vi "Client.vi"() -> ()   [LabVIEW 2025]
uses:
  <vilib>/Utility/miscctls.llb/LVPointTypeDef.ctl
  common/types/network/FieldData.ctl
  common/types/network/FoggedFieldCell.ctl
  server/types/TerrainEnum.ctl
  <vilib>/Utility/miscctls.llb/LVMapReplaceAction.ctl
  2d6ff062-9b47-4ee0-9ab3-b22f700b8ac0.vi
  ClientGlobalVariables.vi
panel:
  out "Network Ready":bool
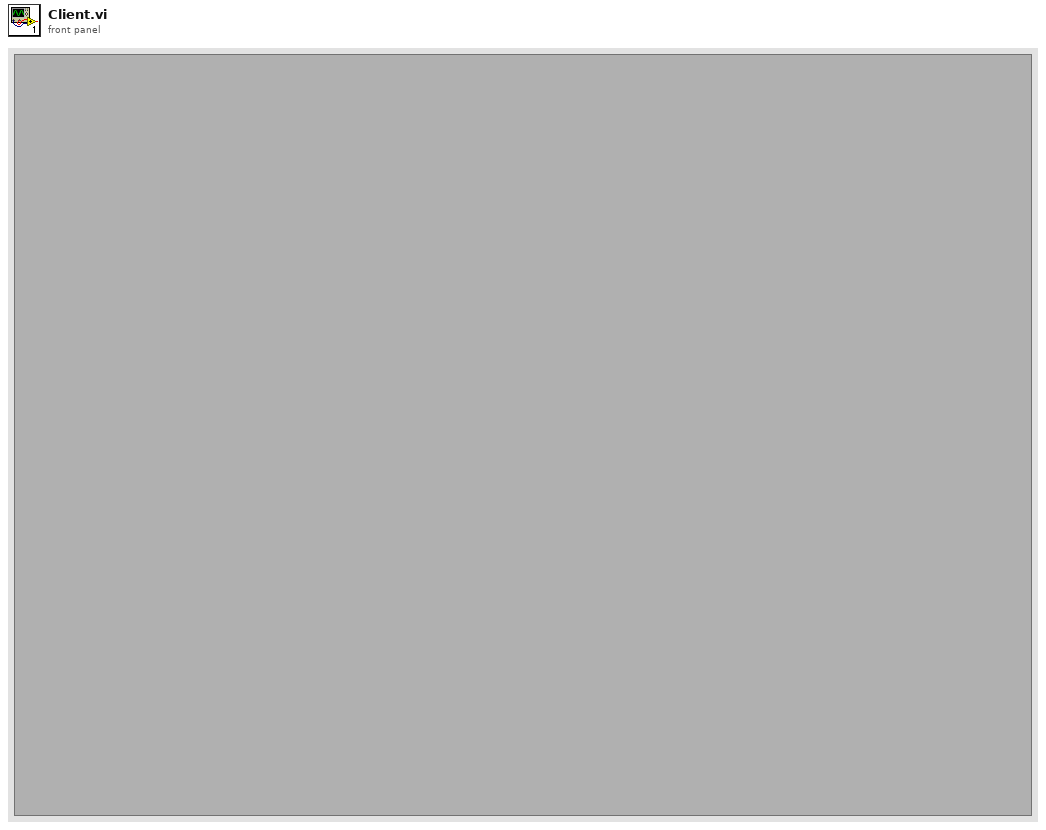
[diagram p1: front panel]
types:
  T1 = cluster{"seconds since 1Jan1904":timestamp, "Data":string}
  T2 = typedef "LVPointTypeDef.ctl" = cluster{"Horizontal":i16, "Vertical":i16}
  T3 = enum16{"Initalize", "Start Menu", "Lobby Menu", "In Game"}
  T4 = cluster{"Action":string, "seconds since 1Jan1904":timestamp, "Data":string}
  T5 = typedef "FieldData.ctl" = cluster{"Round":u32, "FoggedFieldArray":T6[][]}
  T6 = typedef "FoggedFieldCell.ctl" = cluster{"Troops":u32, "Owner":i32, "Terrain":T7, "Fog":bool}
  T7 = typedef "TerrainEnum.ctl" = enum16{"Plain", "Mountain", "City", "General"}
  T8 = map{u32, cluster{"Name":string, "Team":u8, "Ready":bool, "Host":bool, "Alive":bool, "Color":u32, "Lands":set{cluster{"Row":u32, "Column":u32}}, "Army":u32}}
  T9 = cluster{"Name":string, "Team":u8, "Ready":bool, "Host":bool, "Alive":bool, "Color":u32, "Lands":set{cluster{"Row":u32, "Column":u32}}, "Army":u32}
  T10 = typedef "LVMapReplaceAction.ctl" = enum32{"Modify Entry only if found", "Add or Modify Entry", "Delete Entry"}
  T11 = cluster{"ID":u32, "Name":string, "Team":u8, "Ready":bool, "Host":bool, "Alive":bool, "Color":u32, "Lands":set{cluster{"Row":u32, "Column":u32}}, "Army":u32}[]
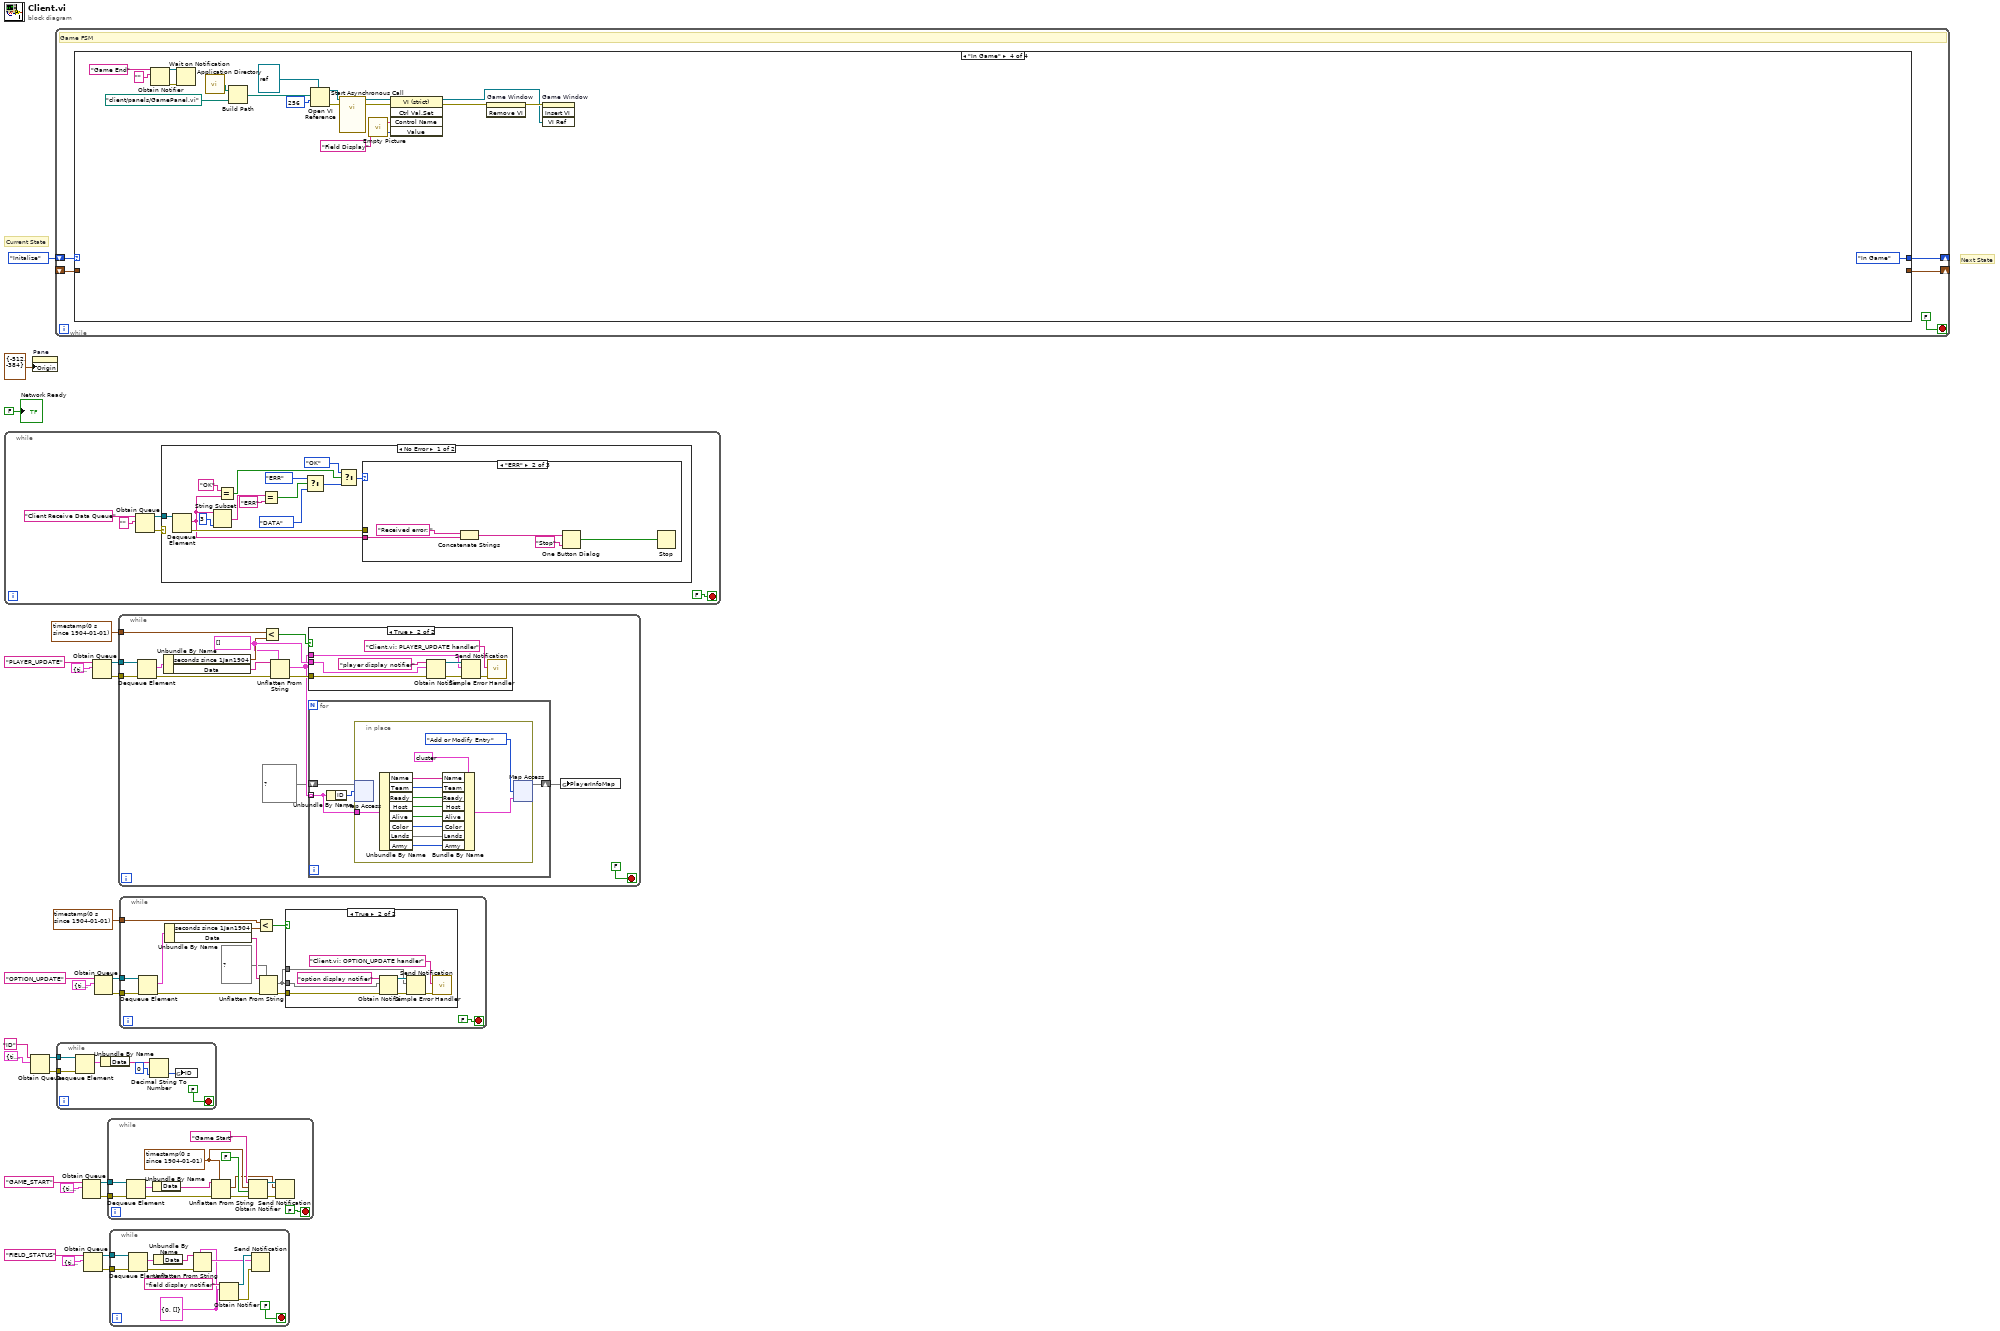
[diagram p0: block diagram]
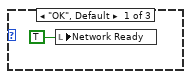
[diagram p4: hidden frame]
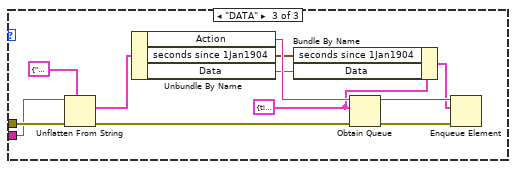
[diagram p5: hidden frame]
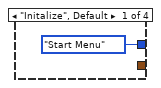
[diagram p7: hidden frame]
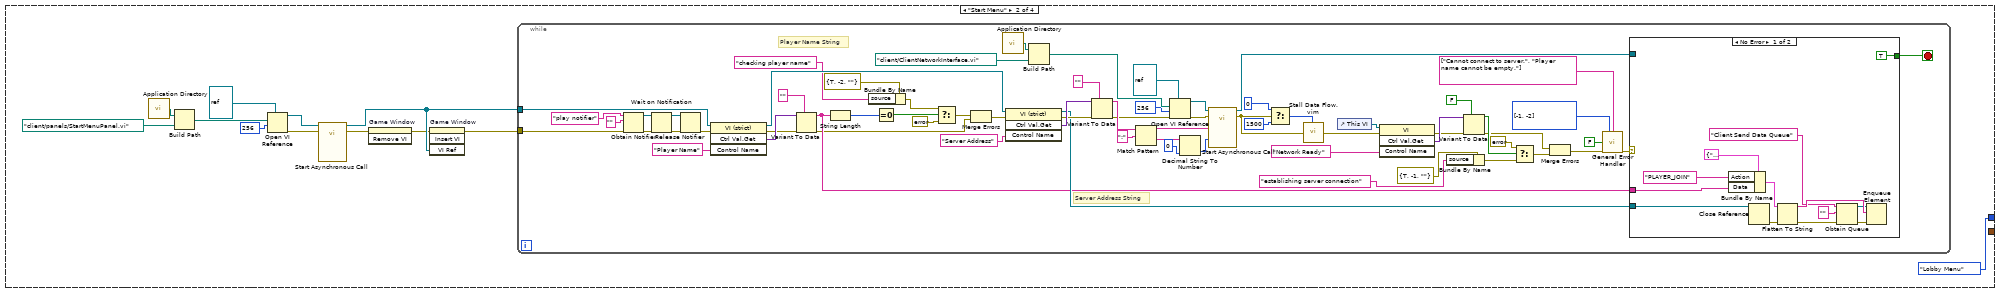
[diagram p8: hidden frame]
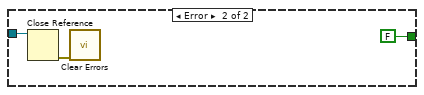
[diagram p9: hidden frame]
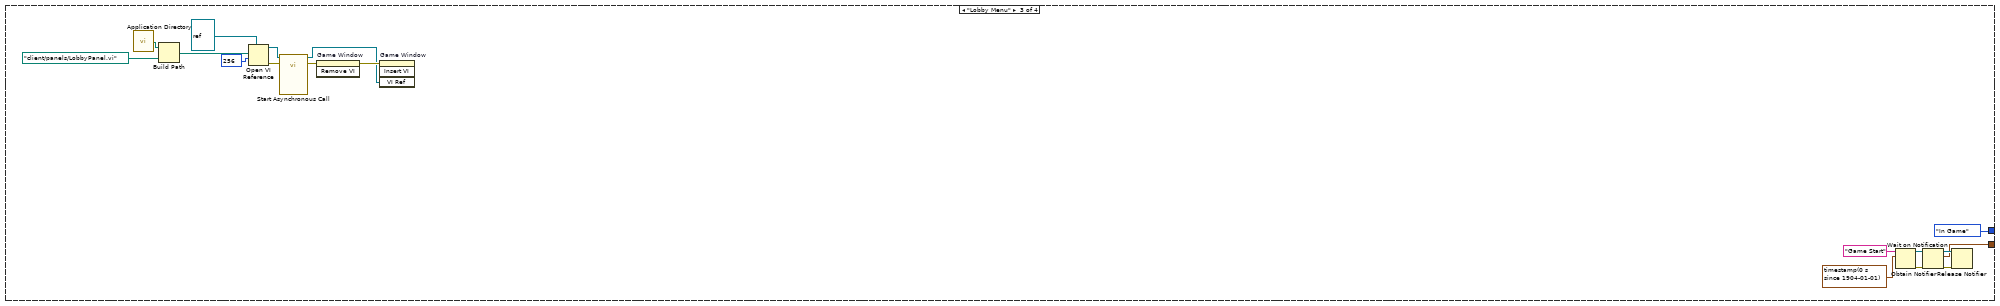
[diagram p10: hidden frame]
diagram:
  # "Current State"
  # "Next State"
  n1 = while {
    stop <- FALSE stop-if-true
    n2 = Obtain Queue(name (unnamed)="Client Receive Data Queue", element data type="") -> (queue out=w28:refnum<queue>, error out=w29:errorcluster)  [unwired: 3 in, 1 out]
    n3 = case shown="No Error" w29 {
      tunnel: w28 -> [w42 _]
      frame No Error {
        n4 = Dequeue Element(queue=w42) -> (element=w38:string, error out=w44:errorcluster)  [unwired: 2 in, 2 out]
        n5 = String Subset(string=w38, length (rest)=3 ("length (rest)")) -> (substring=w35:string)  [unwired: 1 in]
        n6 = Equal?(x="OK", y=w38) -> (x = y?=w41:bool)
        n7 = Equal?(x=w35, y="ERR") -> (x = y?=w36:bool)
        n8 = Select(t=enum16{"OK", "ERR", "DATA"}."ERR", s=w36, f=enum16{"OK", "ERR", "DATA"}."DATA") -> (s? t:f=w39:enum16{"OK", "ERR", "DATA"})
        n9 = Select(t=enum16{"OK", "ERR", "DATA"}."OK", s=w41, f=w39) -> (s? t:f=w31:enum16{"OK", "ERR", "DATA"})
        n10 = case shown="\"ERR\"" w31 {
          tunnel: w44 -> [_ _ w60]
          tunnel: w38 -> [_ w49 w51]
          frame "OK", Default {
            n11 = local write "Network Ready"(TRUE) -> ()
          }
          frame "ERR" {
            n12 = Concatenate Strings("Received error: " ("string"), w49) -> (w48:string)
            n13 = One Button Dialog(message=w48, button name ("OK")="Stop") -> (true=w46:bool)
            n14 = Stop(stop? (T)=w46) -> ()
          }
          frame "DATA" {
            w56 = T1 {"seconds since 1Jan1904"=timestamp(0 s since 1904-01-01), "Data"=""}
            n15 = Unflatten From String(type=T4 {"Action"="", "seconds since 1Jan1904"=timestamp(0 s since 1904-01-01), "Data"=""} ("output cluster"), binary string=w51, error in (no error)=w60) -> (value=w61:T4, error out=w58:errorcluster)  [unwired: 2 in, 1 out]
            n16 = Unbundle By Name(w61) -> ("Action"=w59:string, "seconds since 1Jan1904"=w55:timestamp, "Data"=w54:string)
            n17 = Bundle By Name(cluster=w56, "seconds since 1Jan1904"=w55, "Data"=w54) -> (w53:T1)
            n18 = Obtain Queue(name (unnamed)=w59, element data type=w56, error in (no error)=w58) -> (queue out=w57:refnum<queue>, error out=w52:errorcluster)  [unwired: 2 in, 1 out]
            n19 = Enqueue Element(queue=w57, element=w53, error in (no error)=w52) -> ()  [unwired: 1 in, 3 out]
          }
        }
      }
      frame Error {
      }
    }
  }
  n20 = Obtain Queue(name (unnamed)="ID", element data type=T1 {"seconds since 1Jan1904"=timestamp(0 s since 1904-01-01), "Data"=""}) -> (queue out=w12:refnum<queue>, error out=w13:errorcluster)  [unwired: 3 in, 1 out]
  n21 = property on="Pane" class="Pane"("Origin"=T2 {"Horizontal"=-512, "Vertical"=-384}) -> ()  [unwired: 2 in, 2 out]
  n22 = while {
    shift-right: [w65] -> _
    shift-left: T3."Initalize" -> [w67]
    shift-right: [w64] -> _
    shift-left: _ -> [w63]
    stop <- FALSE stop-if-true
    # "Game FSM"
    n23 = case shown="\"In Game\"" w67 {
      tunnel: [T3."Start Menu" T3."Lobby Menu" T3."In Game" T3."In Game"] -> w65
      tunnel: [_ _ w165 _] -> w64
      tunnel: w63 -> [_ _ _ _]
      frame "Initalize", Default {
      }
      frame "Start Menu" {
        n24 = call <vilib>:"Application Directory.vi"() -> ("Application Directory"=w78:path)
        n25 = Build Path(base path=w78, name or relative path=path "client/panels/StartMenuPanel.vi" ("vi path")) -> (appended path=w79:path)
        n26 = Open VI Reference(type specifier VI Refnum (for type only)=refnum<vi> refnum, vi path=w79, options=256) -> (vi reference=w74:refnum<vi>, error out=w69:errorcluster)  [unwired: 3 in]
        n27 = call-by-ref "Start Asynchronous Call"(reference=w74, error in=w69) -> (reference out=w73:refnum<vi>, error out=w71:errorcluster)  [unwired: 1 in]
        n28 = invoke on="Game Window" class="SubPnl" method="Remove VI"(error in=w71) -> (error out=w70:errorcluster)  [unwired: 2 in, 2 out]
        n29 = invoke on="Game Window" class="SubPnl" method="Insert VI"(error in=w70, "VI Ref"=w73) -> (error out=w77:errorcluster)  [unwired: 2 in, 3 out]
        n30 = while {
          tunnel: w73 -> [w122]
          tunnel: w77 -> [w88]
          stop <- w116 stop-if-true
          # "Server Address String"
          # "Player Name String"
          n31 = Obtain Notifier(name (unnamed)="play notifier", notification data type="", error in (no error)=w88) -> (notifier out=w86:refnum<notifier>, error out=w87:errorcluster)  [unwired: 1 in, 1 out]
          n32 = Wait on Notification(notifier=w86, error in (no error)=w87) -> (notifier out=w83:refnum<notifier>, error out=w82:errorcluster)  [unwired: 2 in, 2 out]
          n33 = Release Notifier(notifier=w83, error in (no error)=w82) -> (error out=w81:errorcluster)  [unwired: 1 in, 2 out]
          n34 = invoke class="VI (strict)" method="Ctrl Val.Get"(reference=w122, error in=w81, "Control Name"="Player Name") -> (reference out=w146:refnum<vi>, error out=w143:errorcluster, "Get Control Value Variant"=w144:variant)  [unwired: 1 in, 1 out]
          n35 = Variant To Data(error in=w143, type="", Variant=w144) -> (data=w117:string, error out=w99:errorcluster)
          n36 = String Length(string=w117) -> (length=w118:i32)
          n37 = Bundle By Name(cluster=errorcluster {"status"=TRUE, "code"=-2, "source"=""} ("error constant"), "source"="checking player name") -> (w112:errorcluster)
          n38 = Equal To 0?(x=w118) -> (x = 0?=w115:bool)
          n39 = Select(t=w112, s=w115, f=errorcluster {"status"=FALSE, "code"=0, "source"=""}) -> (s? t:f=w101:errorcluster)
          n40 = Merge Errors(w101, w99) -> (w100:errorcluster)
          n41 = call <vilib>:"Application Directory.vi"() -> ("Application Directory"=w132:path)
          n42 = invoke class="VI (strict)" method="Ctrl Val.Get"(reference=w146, error in=w100, "Control Name"="Server Address") -> (reference out=w121:refnum<vi>, error out=w139:errorcluster, "Get Control Value Variant"=w141:variant)  [unwired: 1 in, 1 out]
          n43 = Build Path(base path=w132, name or relative path=path "client/ClientNetworkInterface.vi" ("vi path")) -> (appended path=w133:path)
          n44 = Variant To Data(error in=w139, type="", Variant=w141) -> (data=w137:string, error out=w128:errorcluster)
          n45 = Match Pattern(string=w137, regular expression=":") -> (before substring=w120:string, after substring=w136:string)  [unwired: 1 in, 2 out]
          n46 = Open VI Reference(type specifier VI Refnum (for type only)=refnum<vi> refnum, vi path=w133, options=256, error in (no error)=w128) -> (vi reference=w127:refnum<vi>, error out=w129:errorcluster)  [unwired: 2 in]
          n47 = Decimal String To Number(string=w136, default (0L)=u16 0 ("default (0 I32)")) -> (number=w119:u16)  [unwired: 1 in, 1 out]
          n48 = call-by-ref "Start Asynchronous Call"(reference=w127, error in=w129, "Server Port"=w119, "Server Address"=w120) -> (reference out=w92:refnum<vi>, error out=w90:errorcluster)
          n49 = Select(t=u32 0 ("milliseconds to wait"), s=w90, f=u32 1500) -> (s? t:f=w89:u32)
          n50 = call "Stall Data Flow.vim"("value in"=w90, "milliseconds to wait"=w89) -> ("value out"=w91:errorcluster)  [unwired: 1 out]
          n51 = control-ref of="This VI"() -> (w93:refnum<vi>)
          n52 = invoke class="VI" method="Ctrl Val.Get"(reference=w93, error in=w91, "Control Name"="Network Ready") -> (error out=w123:errorcluster, "Get Control Value Variant"=w125:variant)  [unwired: 1 in, 2 out]
          n53 = Bundle By Name(cluster=errorcluster {"status"=TRUE, "code"=-1, "source"=""} ("f"), "source"="establishing server connection") -> (w108:errorcluster)
          n54 = Variant To Data(error in=w123, type=FALSE, Variant=w125) -> (data=w110:bool, error out=w103:errorcluster)
          n55 = Select(t=errorcluster {"status"=FALSE, "code"=0, "source"=""}, s=w110, f=w108) -> (s? t:f=w104:errorcluster)
          n56 = Merge Errors(w103, w104) -> (w105:errorcluster)
          n57 = call <vilib>:"General Error Handler.vi"("[user-defined codes]"=i32[] [-1, -2], "[user-defined descriptions]"=string[] ["Cannot connect to server.", "Player name cannot be empty."], "search ni.com link visible?(T)"=FALSE, "error in (no error)"=w105) -> ("error out"=w111:errorcluster)  [unwired: 7 in, 4 out]
          n58 = case shown="No Error" w111 {
            tunnel: w121 -> [w160 _]
            tunnel: w117 -> [w157 _]
            tunnel: [TRUE FALSE] -> w116
            tunnel: w92 -> [_ w162]
            frame No Error {
              n59 = Bundle By Name(cluster=cluster{"Action":string, "Data":string} {"Action"="", "Data"=""} ("CommandCluster"), "Action"="PLAYER_JOIN", "Data"=w157) -> (w156:cluster{"Action":string, "Data":string})
              n60 = Close Reference(reference=w160) -> (error out=w155:errorcluster)  [unwired: 1 in]
              n61 = Flatten To String(anything=w156, error in (no error)=w155) -> (data string=w154:string, error out=w149:errorcluster)  [unwired: 2 in, 1 out]
              n62 = Obtain Queue(name (unnamed)="Client Send Data Queue", element data type="", error in (no error)=w149) -> (queue out=w150:refnum<queue>, error out=w148:errorcluster)  [unwired: 2 in, 1 out]
              n63 = Enqueue Element(queue=w150, element=w154, error in (no error)=w148) -> ()  [unwired: 1 in, 3 out]
            }
            frame Error {
              n64 = Close Reference(reference=w162) -> (error out=w161:errorcluster)  [unwired: 1 in]
              n65 = call <vilib>:"Clear Errors.vi"("error in (no error)"=w161) -> ()  [unwired: 5 in, 2 out]
            }
          }
        }
      }
      frame "Lobby Menu" {
        n66 = call <vilib>:"Application Directory.vi"() -> ("Application Directory"=w178:path)
        n67 = Build Path(base path=w178, name or relative path=path "client/panels/LobbyPanel.vi" ("vi path")) -> (appended path=w179:path)
        n68 = Open VI Reference(type specifier VI Refnum (for type only)=refnum<vi> refnum, vi path=w179, options=256) -> (vi reference=w176:refnum<vi>, error out=w164:errorcluster)  [unwired: 3 in]
        n69 = call-by-ref "Start Asynchronous Call"(reference=w176, error in=w164) -> (reference out=w173:refnum<vi>, error out=w175:errorcluster)  [unwired: 1 in]
        n70 = invoke on="Game Window" class="SubPnl" method="Remove VI"(error in=w175) -> (error out=w174:errorcluster)  [unwired: 2 in, 2 out]
        n71 = invoke on="Game Window" class="SubPnl" method="Insert VI"(error in=w174, "VI Ref"=w173) -> ()  [unwired: 2 in, 4 out]
        n72 = Obtain Notifier(name (unnamed)="Game Start", notification data type=timestamp(0 s since 1904-01-01) ("x+y")) -> (notifier out=w170:refnum<notifier>, error out=w169:errorcluster)  [unwired: 2 in, 1 out]
        n73 = Wait on Notification(notifier=w170, error in (no error)=w169) -> (notifier out=w168:refnum<notifier>, notification=w165:timestamp, error out=w167:errorcluster)  [unwired: 2 in, 1 out]
        n74 = Release Notifier(notifier=w168, error in (no error)=w167) -> ()  [unwired: 1 in, 3 out]
      }
      frame "In Game" {
        n75 = Obtain Notifier(name (unnamed)="Game End", notification data type="") -> (notifier out=w191:refnum<notifier>, error out=w190:errorcluster)  [unwired: 2 in, 1 out]
        n76 = Wait on Notification(notifier=w191, error in (no error)=w190) -> ()  [unwired: 2 in, 4 out]
        n77 = call <vilib>:"Application Directory.vi"() -> ("Application Directory"=w197:path)
        n78 = Build Path(base path=w197, name or relative path=path "client/panels/GamePanel.vi" ("vi path")) -> (appended path=w198:path)
        n79 = Open VI Reference(type specifier VI Refnum (for type only)=refnum<vi> refnum, vi path=w198, options=256) -> (vi reference=w188:refnum<vi>, error out=w193:errorcluster)  [unwired: 3 in]
        n80 = call-by-ref "Start Asynchronous Call"(reference=w188, error in=w193) -> (reference out=w183:refnum<vi>, error out=w185:errorcluster)  [unwired: 1 in]
        n81 = call "Empty Picture"() -> ("empty picture"=w186:picture)
        n82 = invoke class="VI (strict)" method="Ctrl Val.Set"(reference=w183, error in=w185, "Control Name"="Field Display", "Value"=w186) -> (reference out=w182:refnum<vi>, error out=w184:errorcluster)  [unwired: 1 in, 3 out]
        n83 = invoke on="Game Window" class="SubPnl" method="Remove VI"(error in=w184) -> (error out=w195:errorcluster)  [unwired: 2 in, 2 out]
        n84 = invoke on="Game Window" class="SubPnl" method="Insert VI"(error in=w195, "VI Ref"=w182) -> ()  [unwired: 2 in, 4 out]
      }
    }
  }
  n85 = while {
    tunnel: w12 -> [w207]
    tunnel: w13 -> [w206]
    stop <- FALSE stop-if-true
    n86 = Dequeue Element(queue=w207, error in (no error)=w206) -> (element=w205:T1)  [unwired: 1 in, 3 out]
    n87 = Unbundle By Name(w205) -> ("Data"=w203:string)
    n88 = Decimal String To Number(string=w203, default (0L)=u32 0 ("ID")) -> (number=w201:u32)  [unwired: 1 in, 1 out]
    n89 = global write "ClientGlobalVariables.vi" "ID"(w201) -> ()
  }
  n90 = Obtain Queue(name (unnamed)="GAME_START", element data type=T1 {"seconds since 1Jan1904"=timestamp(0 s since 1904-01-01), "Data"=""}) -> (queue out=w6:refnum<queue>, error out=w7:errorcluster)  [unwired: 3 in, 1 out]
  n91 = Obtain Queue(name (unnamed)="FIELD_STATUS" ("Action"), element data type=T1 {"seconds since 1Jan1904"=timestamp(0 s since 1904-01-01), "Data"=""}) -> (queue out=w3:refnum<queue>, error out=w4:errorcluster)  [unwired: 3 in, 1 out]
  n92 = Obtain Queue(name (unnamed)="PLAYER_UPDATE", element data type=T1 {"seconds since 1Jan1904"=timestamp(0 s since 1904-01-01), "Data"=""}) -> (queue out=w23:refnum<queue>, error out=w22:errorcluster)  [unwired: 3 in, 1 out]
  n93 = Obtain Queue(name (unnamed)="OPTION_UPDATE", element data type=T1 {"seconds since 1Jan1904"=timestamp(0 s since 1904-01-01), "Data"=""}) -> (queue out=w18:refnum<queue>, error out=w17:errorcluster)  [unwired: 3 in, 1 out]
  n94 = while {
    tunnel: w6 -> [w220]
    tunnel: w7 -> [w219]
    stop <- FALSE stop-if-true
    w212 = timestamp(0 s since 1904-01-01) ("x+y")
    n95 = Dequeue Element(queue=w220, error in (no error)=w219) -> (element=w217:T1, error out=w215:errorcluster)  [unwired: 1 in, 2 out]
    n96 = Unbundle By Name(w217) -> ("Data"=w216:string)
    n97 = Unflatten From String(type=w212, binary string=w216, error in (no error)=w215) -> (value=w209:timestamp, error out=w211:errorcluster)  [unwired: 2 in, 1 out]
    n98 = Obtain Notifier(name (unnamed)="Game Start", notification data type=w212, create if not found? (T)=FALSE, error in (no error)=w211) -> (notifier out=w210:refnum<notifier>, error out=w208:errorcluster)  [unwired: 1 out]
    n99 = Send Notification(notification=w209, notifier=w210, error in (no error)=w208) -> ()  [unwired: 2 out]
  }
  n100 = while {
    tunnel: w3 -> [w231]
    tunnel: w4 -> [w230]
    stop <- FALSE stop-if-true
    w221 = T5 {"Round"=0, "FoggedFieldArray"=[]} ("CellInfo 2")
    n101 = Dequeue Element(queue=w231, error in (no error)=w230) -> (element=w229:T1, error out=w223:errorcluster)  [unwired: 1 in, 2 out]
    n102 = Unbundle By Name(w229) -> ("Data"=w224:string)
    n103 = Unflatten From String(type=w221, binary string=w224, error in (no error)=w223) -> (value=w222:T5)  [unwired: 2 in, 2 out]
    n104 = Obtain Notifier(name (unnamed)="field display notifier", notification data type=w221) -> (notifier out=w226:refnum<notifier>, error out=w225:errorcluster)  [unwired: 2 in, 1 out]
    n105 = Send Notification(notification=w222, notifier=w226, error in (no error)=w225) -> ()  [unwired: 2 out]
  }
  n106 = while {
    tunnel: w23 -> [w245]
    tunnel: w22 -> [w244]
    tunnel: timestamp(0 s since 1904-01-01) ("seconds since 1Jan1904") -> [w241]
    stop <- FALSE stop-if-true
    w235 = T11 [] ("PlayerInfoArray")
    n107 = Dequeue Element(queue=w245, error in (no error)=w244) -> (element=w243:T1, error out=w238:errorcluster)  [unwired: 1 in, 2 out]
    n108 = Unbundle By Name(w243) -> ("seconds since 1Jan1904"=w242:timestamp, "Data"=w239:string)
    n109 = Less?(x=w241, y=w242) -> (x < y?=w240:bool)
    n110 = Unflatten From String(type=w235, binary string=w239, error in (no error)=w238) -> (value=w234:T11, error out=w236:errorcluster)  [unwired: 2 in, 1 out]
    n111 = case shown="True" w240 {
      tunnel: w234 -> [_ w265]
      tunnel: w236 -> [_ w263]
      tunnel: w235 -> [_ w266]
      frame False {
      }
      frame True {
        n112 = Obtain Notifier(name (unnamed)="player display notifier", notification data type=w266, error in (no error)=w263) -> (notifier out=w269:refnum<notifier>, error out=w264:errorcluster)  [unwired: 1 in, 1 out]
        n113 = Send Notification(notification=w265, notifier=w269, error in (no error)=w264) -> (error out=w268:errorcluster)  [unwired: 1 out]
        n114 = call <vilib>:"Simple Error Handler.vi"("error source (\" \")"="Client.vi: PLAYER_UPDATE handler" ("error source (\" \")"), "error in (no error)"=w268) -> ()  [unwired: 3 in, 5 out]
      }
    }
    n115 = for {
      tunnel: w234 -> [w247] mode=indexing
      shift-right: [w246] -> w232
      shift-left: T8 {} ("PlayerInfoMap") -> [w249]
      n116 = Unbundle By Name(w247) -> ("ID"=w248:u32)
      n117 = in-place {
        in-place-border: w247 -> [w259]
        n118 = in-place-map #1(w249, w248) -> ()  [unwired: 1 in, 2 out]
        n119 = Unbundle By Name(w259) -> ("Name"=w258:string, "Team"=w257:u8, "Ready"=w256:bool, "Host"=w255:bool, "Alive"=w254:bool, "Color"=w253:u32, "Lands"=w252:set{cluster{"Row":u32, "Column":u32}}, "Army"=w251:u32)
        n120 = Bundle By Name(cluster=T9 {"Name"="", "Team"=0, "Ready"=FALSE, "Host"=FALSE, "Alive"=FALSE, "Color"=0, "Lands"={}, "Army"=0} ("value"), "Name"=w258, "Team"=w257, "Ready"=w256, "Host"=w255, "Alive"=w254, "Color"=w253, "Lands"=w252, "Army"=w251) -> (w250:T9)
        n121 = in-place-map #1(w250, LVMapReplaceAction."Add or Modify Entry" ("action")) -> (w246:T8)  [unwired: 2 out]
      }
    }
    n122 = global write "ClientGlobalVariables.vi" "PlayerInfoMap"(w232) -> ()
  }
  n123 = while {
    tunnel: w18 -> [w281]
    tunnel: w17 -> [w280]
    tunnel: timestamp(0 s since 1904-01-01) ("seconds since 1Jan1904") -> [w277]
    stop <- FALSE stop-if-true
    n124 = Dequeue Element(queue=w281, error in (no error)=w280) -> (element=w279:T1, error out=w274:errorcluster)  [unwired: 1 in, 2 out]
    n125 = Unbundle By Name(w279) -> ("seconds since 1Jan1904"=w278:timestamp, "Data"=w275:string)
    n126 = Less?(x=w277, y=w278) -> (x < y?=w276:bool)
    n127 = Unflatten From String(type=map{string, i32} {} ("Options"), binary string=w275, error in (no error)=w274) -> (value=w270:map{string, i32}, error out=w272:errorcluster)  [unwired: 2 in, 1 out]
    n128 = case shown="True" w276 {
      tunnel: w272 -> [_ w283]
      tunnel: w270 -> [_ w285]
      tunnel: w270 -> [_ w284]
      frame False {
      }
      frame True {
        n129 = Obtain Notifier(name (unnamed)="option display notifier", notification data type=w285, error in (no error)=w283) -> (notifier out=w288:refnum<notifier>, error out=w289:errorcluster)  [unwired: 1 in, 1 out]
        n130 = Send Notification(notification=w284, notifier=w288, error in (no error)=w289) -> (error out=w287:errorcluster)  [unwired: 1 out]
        n131 = call <vilib>:"Simple Error Handler.vi"("error source (\" \")"="Client.vi: OPTION_UPDATE handler" ("error source (\" \")"), "error in (no error)"=w287) -> ()  [unwired: 3 in, 5 out]
      }
    }
  }
  "Network Ready" <- FALSE ("Network Ready")
